vi "modbusTCPSlaveDriver.vi"(6 "Modbus Driver Selector Enum":T3, 8 "Error In":errorcluster, 9 "Read Modbus Register":T1, 10 "Write Single Register Modbus":T2, 11 "Port (502)":u16) -> (0 "Error Out":errorcluster, 3 "Register Value":u16[](array[numeric]))   [LabVIEW 2018]
uses:
  controls/modbusDriverSelectorEnum.ctl
  controls/writeSingleRegisterModbusCluster.ctl
  controls/readRegisterModbusCluster.ctl
  <vilib>/NI/Modbus Library/API/Slave/Modbus Slave.lvclass
  C:/Program Files (x86)/National Instruments/LabVIEW 2018/vi.lib/NI/Modbus Library/API/Modbus API.lvclass
  <vilib>/NI/Modbus Library/API/Wrapper/Create TCP Slave.vi
  <vilib>/NI/Modbus Library/API/Modbus API.lvclass
  <vilib>/NI/Modbus Library/API/Wrapper/API Main.lvlib
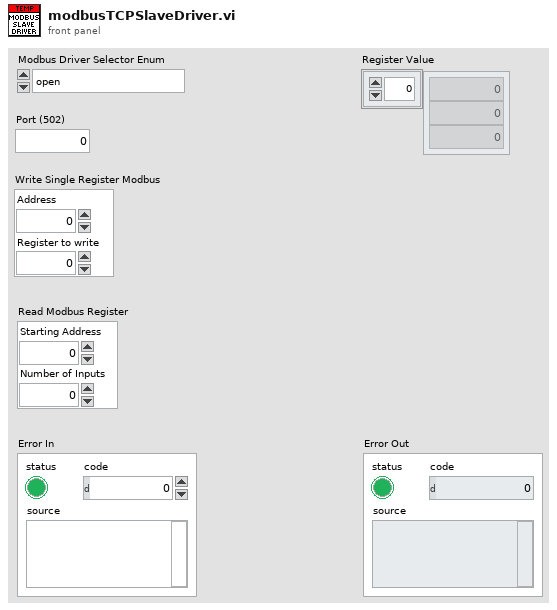
[diagram p1: front panel]
types:
  T1 = typedef "readRegisterModbusCluster.ctl" = cluster{"Starting Address":u16, "Number of Inputs":u16}
  T2 = typedef "writeSingleRegisterModbusCluster.ctl" = cluster{"Address":u16, "Register to write":u16}
  T3 = typedef "modbusDriverSelectorEnum.ctl" = enum16{"open", "write single holding registers", "read holding registers", "close"}
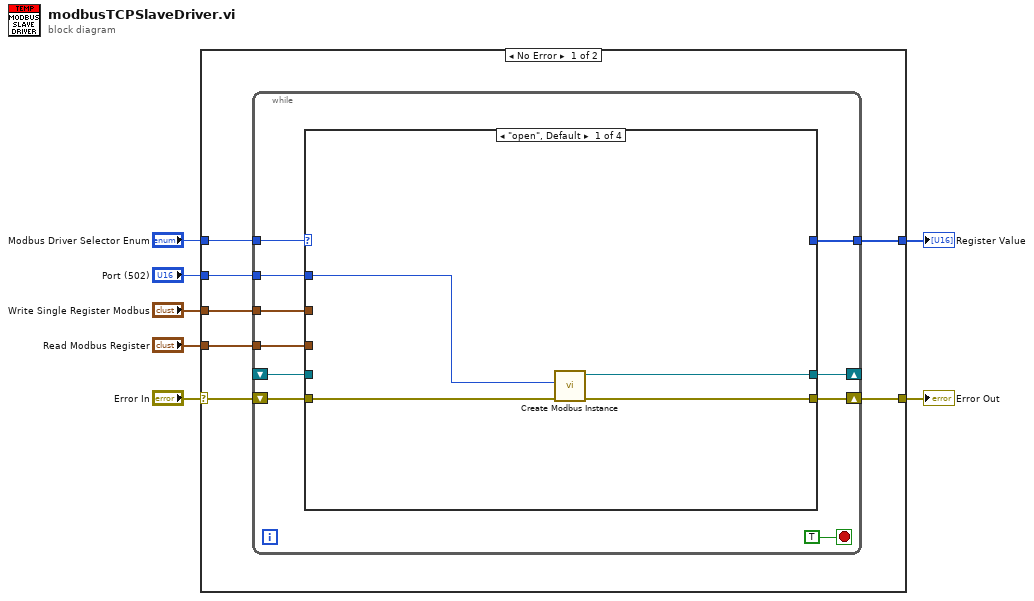
[diagram p0: block diagram]
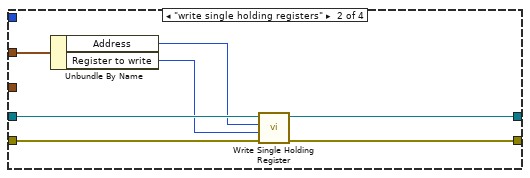
[diagram p2: hidden frame]
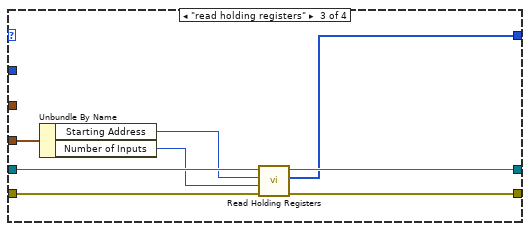
[diagram p3: hidden frame]
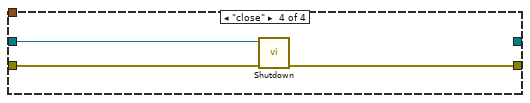
[diagram p4: hidden frame]
diagram:
  n1 = case shown="No Error" "Error In" {
    selector: "Error In" -> [w14 w47]
    tunnel: [w13 w47] -> w5
    tunnel: "Modbus Driver Selector Enum" -> [w12 _]
    tunnel: [w11 _] -> w4
    tunnel: "Read Modbus Register" -> [w10 _]
    tunnel: "Write Single Register Modbus" -> [w9 _]
    tunnel: "Port (502)" -> [w8 _]
    frame No Error {
      n2 = while {
        tunnel: w12 -> [w22]
        shift-right: [w23] -> w13
        shift-left: w14 -> [w24]
        shift-right: [w21] -> _
        shift-left: _ -> [w20]
        tunnel: [w18] -> w11
        tunnel: w10 -> [w17]
        tunnel: w9 -> [w16]
        tunnel: w8 -> [w15]
        stop <- TRUE stop-if-true
        n3 = case shown="\"open\", Default" w22 {
          tunnel: w24 -> [w27 w34 w42 w45]
          tunnel: [w28 w35 w43 w46] -> w23
          tunnel: [w26 w33 w41 _] -> w21
          tunnel: w20 -> [_ w32 w40 w44]
          tunnel: [_ _ w39 _] -> w18
          tunnel: w17 -> [_ _ w38 _]
          tunnel: w16 -> [_ w31 _ _]
          tunnel: w15 -> [w25 _ _ _]
          frame "open", Default {
            n4 = call-poly <vilib>:"Create Modbus Instance.vi"("error in"=w27, "port (502)"=w25) -> ("error out"=w28:errorcluster, "TCP slave instance"=w26:refnum<class "Modbus Slave.lvclass">)  [unwired: 8 in]
          }
          frame "write single holding registers" {
            n5 = Unbundle By Name(w31) -> ("Address"=w30:u16, "Register to write"=w29:u16)
            n6 = call-dynamic "Write Single Holding Register.vi"("error in"=w34, "register to write"=w29, "address"=w30, "Modbus instance in"=w32) -> ("error out"=w35:errorcluster, "Modbus instance out"=w33:refnum<class "Modbus API.lvclass">)  [unwired: 6 in]
          }
          frame "read holding registers" {
            n7 = Unbundle By Name(w38) -> ("Starting Address"=w37:u16, "Number of Inputs"=w36:u16)
            n8 = call-dynamic "Read Holding Registers.vi"("error in"=w42, "number of inputs"=w36, "starting address"=w37, "Modbus instance in"=w40) -> ("error out"=w43:errorcluster, "register values"=w39:u16[], "Modbus instance out"=w41:refnum<class "Modbus API.lvclass">)  [unwired: 5 in]
          }
          frame "close" {
            n9 = call-dynamic "Shutdown.vi"("error in"=w45, "Modbus instance in"=w44) -> ("error out"=w46:errorcluster)  [unwired: 9 in]
          }
        }
      }
    }
    frame Error {
    }
  }
  "Error Out" <- w5
  "Register Value" <- w4
